vi "get_voltage_and_current_set_high_limit.vi"(8 "error in":errorcluster, 11 "VISA resource name":refnum<visa-resource-name>="COM1") -> (0 "error out":errorcluster, 3 "Response":string)   [LabVIEW 2020]
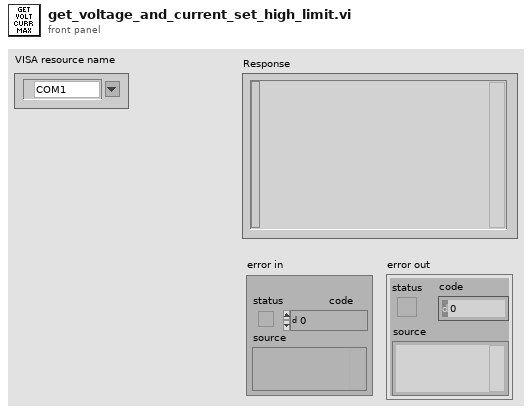
[diagram p1: front panel]
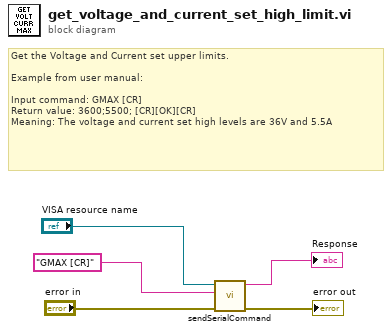
[diagram p0: block diagram]
diagram:
  # "Get the Voltage and Current set upper limits.\n\nExample from user manual:\n\nInput command: GMAX [CR]\nReturn value: 3600;5500; [CR][OK][CR]\nMeaning: The voltage and current set high levels are 36V and 5.5A"
  n1 = call "sendSerialCommand.vi"("error in (no error)"="error in", "Command"="GMAX [CR]", "VISA resource name"="VISA resource name") -> ("error out"=→"error out":errorcluster, "Response"=→"Response":string)  [unwired: 7 in]
